vi "Add DataTable to DataSet.vi"(8 "error in (no error)":errorcluster caption="错误输入（无错误）", 10 "Data Grid VIEW.lvlib:DataTable.lvclass":refnum<class "DataTable.lvclass">, 11 "DataSet 输入":refnum<class "DataSet.lvclass"> caption="DNL_LabVIEW Object in") -> (0 "error out":errorcluster caption="错误输出", 2 "DataTable输出":refnum<class "DataTable.lvclass">, 3 "DataSet 输出":refnum<class "DataSet.lvclass"> caption="DNL_LabVIEW Object out")   [LabVIEW 2012, in "Data Grid VIEW.lvlib" / "DataSet.lvclass"]
uses:
  DataSet.lvclass
  Data Table/DataTable.lvclass
  Data Table/DataTable.lvclass/DataTable.ctl
  DataSet.lvclass/DataSet.ctl
  System.Data
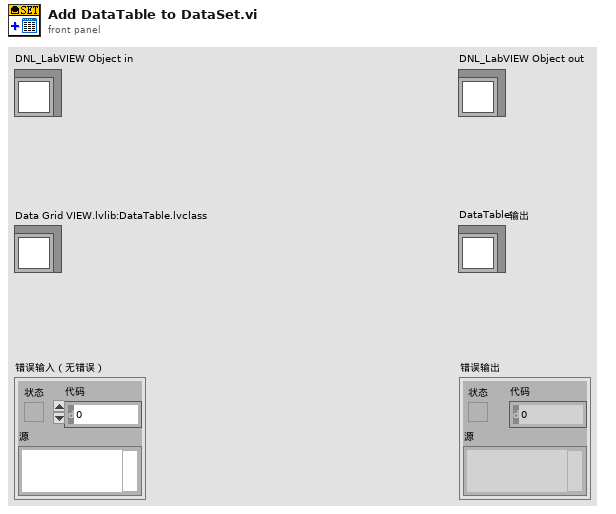
[diagram p1: front panel]
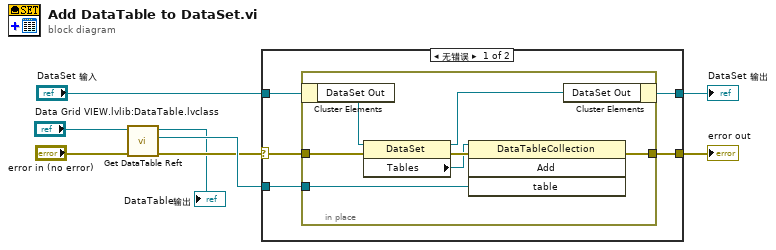
[diagram p0: block diagram]
diagram:
  n1 = call "Get DataTable Reft.vi"("error in (no error)"="error in (no error)", "DataTable输入"="Data Grid VIEW.lvlib:DataTable.lvclass") -> ("error out"=w2:errorcluster, "DataTable"=w4:refnum<k24>, "DataTable输出"=→"DataTable输出":refnum<class "DataTable.lvclass">)  [unwired: 7 in]
  n2 = case shown="无错误" w2 {
    selector: w2 -> [w12 w22]
    tunnel: [w10 w22] -> w8
    tunnel: [w9 w21] -> w6
    tunnel: "DataSet 输入" -> [w13 w21]
    tunnel: w4 -> [w11 _]
    frame No Error {
      n3 = in-place {
        in-place-border: w12 -> [w17]
        in-place-border: w11 -> [w16]
        in-place-border: [w15] -> w10
        n4 = in-place-cluster #1(w13) -> ("DataSet Out"=w18:refnum<k24>)
        n5 = property class="DataSet"(reference=w18, error in=w17) -> (reference out=w14:refnum<k24>, error out=w20:errorcluster, "Tables"=w19:refnum<k24>)
        n6 = invoke class="DataTableCollection" method="Add"(reference=w19, error in=w20, "table"=w16) -> (error out=w15:errorcluster)  [unwired: 1 in, 3 out]
        n7 = in-place-cluster #1("DataSet Out"=w14) -> (w9:refnum<class "DataSet.lvclass">)
      }
    }
    frame Error {
    }
  }
  "error out" <- w8
  "DataSet 输出" <- w6
